vi "ARP-Parse.vi"(11 "Frame (in)":u8[](array[numeric])=[0, 1, 8, 0, 6, 4, 0, 1, 0, 35, 38, 182, 175, 53, 192, 168, 1, 200, 0, 0, 0, 0, 0, 0, 192, 168, 1, 201, 0, 0, 0, 0, 0, 0, 0, 0, 0, 0, 0, 0, 0, 0, 0, 0, 0, 0] format="%02x") -> (1 "Target":cluster{"THA":u8[], "TPA":u8[]}={"THA"=[0, 0, 0, 0, 0, 0], "TPA"=[192, 168, 1, 201]} {"THA" format="%02x"}, 2 "Sender":cluster{"SHA":u8[], "SPA":u8[]}={"SHA"=[0, 35, 38, 182, 175, 53], "SPA"=[192, 168, 1, 200]} {"SHA" format="%02x"}, 3 "Header":T1={"HTYPE"=1, "PTYPE"=2048, "HLEN"=6, "PLEN"=4, "OPER"=1})   [LabVIEW 2018]
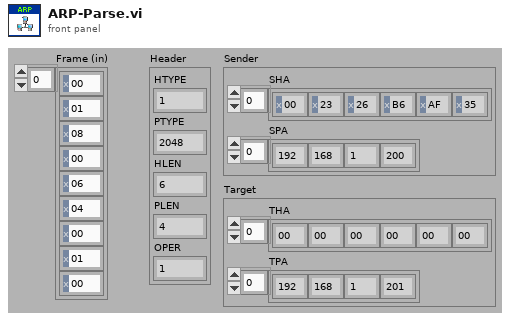
[diagram p1: front panel]
types:
  T1 = cluster{"HTYPE":u16, "PTYPE":u16, "HLEN":u8, "PLEN":u8, "OPER":u16}
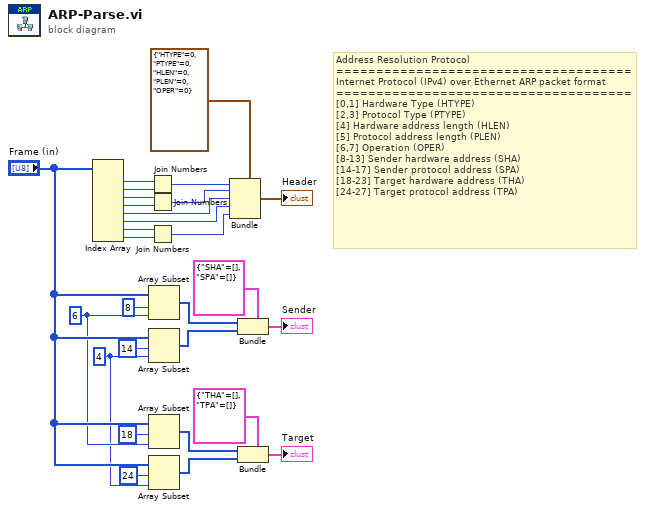
[diagram p0: block diagram]
diagram:
  w13 = 4 ("length")
  w14 = 6 ("length")
  # "Address Resolution Protocol\n=====================================\nInternet Protocol (IPv4) over Ethernet ARP packet format\n===================================== \n[0,1] Hardware Type (HTYPE)\n[2,3] Protocol Type (PTYPE)\n[4] Hardware address length (HLEN)\n[5] Protocol address length (PLEN)\n[6,7] Operation (OPER)\n[8-13] Sender hardware address (SHA)\n[14-17] Sender protocol address (SPA)\n[18-23] Target hardware address (THA)\n[24-27] Target protocol address (TPA)"
  n1 = Index Array(array="Frame (in)") -> (element #1=w25:u8, element #2=w26:u8, element #3=w27:u8, element #4=w28:u8, element #5=w21:u8, element #6=w20:u8, element #7=w16:u8, element #8=w17:u8)  [unwired: 8 in]
  n2 = Join Numbers(hi=w25, lo=w26) -> ((hi.lo)=w24:u16)
  n3 = Join Numbers(hi=w27, lo=w28) -> ((hi.lo)=w22:u16)
  n4 = Join Numbers(hi=w16, lo=w17) -> ((hi.lo)=w15:u16)
  n5 = Array Subset(array="Frame (in)", index=8, length=w14) -> (w12:u8[])
  n6 = Array Subset(array="Frame (in)", index=14, length=w13) -> (w11:u8[])
  n7 = Array Subset(array="Frame (in)", index=18, length=w14) -> (w7:u8[])
  n8 = Array Subset(array="Frame (in)", index=24, length=w13) -> (w6:u8[])
  n9 = Bundle(cluster=T1 {"HTYPE"=0, "PTYPE"=0, "HLEN"=0, "PLEN"=0, "OPER"=0}, "HTYPE"=w24, "PTYPE"=w22, "HLEN"=w21, "PLEN"=w20, "OPER"=w15) -> (→"Header":T1)
  n10 = Bundle(cluster=cluster{"SHA":u8[], "SPA":u8[]} {"SHA"=[], "SPA"=[]}, "SHA"=w12, "SPA"=w11) -> (→"Sender":cluster{"SHA":u8[], "SPA":u8[]})
  n11 = Bundle(cluster=cluster{"THA":u8[], "TPA":u8[]} {"THA"=[], "TPA"=[]}, "THA"=w7, "TPA"=w6) -> (→"Target":cluster{"THA":u8[], "TPA":u8[]})
